vi "Sequence.Test.NextStep.vi"(8 "error in":errorcluster, 11 "Data in":T7={"BeginTS"=timestamp(0 s since 1904-01-01), "EndTS"=timestamp(0 s since 1904-01-01), "State"=enum."Init", "Status.Work"=enum."-", "Status.Process"=enum."-", "Status.Home"=enum."-", "Status.Wabco"=enum."-", "Status.Client"=enum."-", "BreakReason"=enum."-", "BreakSource"=enum."-", "DoorLock"=FALSE, "Status.Prod"=[], "UserAction"={"Stop"=FALSE, "Pause"=FALSE, "Next"=FALSE}, "UserData"={"GuiMode"=enum."Process", "Test"={"IgnoreResults"=FALSE, "IgnoreImages"=FALSE, "ServiceMode"=FALSE}, "ContinueOrder"=FALSE}, "Error"={"status"=FALSE, "code"=0, "source"=""}, "Code"={"Ready"=FALSE, "DoubleOrder"=FALSE, "OrderDone"=FALSE, "AllowSingleSlot"=FALSE, "CheckDM"=FALSE, "ThresholdA"=0, "ThresholdB"=0, "Plate"=enum."Wabco", "ImgPath"=path "", "Variant"={"State"=enum."Init", "ImgPath"=path "", "WabcoPlate"="", "WabcoProduct"="", "ClientProduct"="", "ClientPlate"="", "TotalQuantity"=0, "OrderQuantity"=0, "Serial"=0, "Wabco"={"LaserJob"="", "AdditionalTxt"="037", "FactoryCode"="", "RevID"=0, "ForkID"=0, "FailuresLimit"=0, "GlobalCnt"=0, "ScannerProgram"=0, "SerialFormat"=enum."6 dig", "CoordA"={"X"=0.0, "Y"=0.0, "Angle"=0.0}, "CoordB"={"X"=0.0, "Y"=0.0, "Angle"=0.0}, "DMCconfig"=0}, "Client"={"LaserJob"="", "AdditionalTxt"="", "FactoryCode"="037", "RevID"=0, "ForkID"=0, "FailuresLimit"=0, "GlobalCnt"=0, "ScannerProgram"=0, "SerialFormat"=enum."6 dig", "CoordA"={"X"=0.0, "Y"=0.0, "Angle"=0.0}, "CoordB"={"X"=0.0, "Y"=0.0, "Angle"=0.0}, "DMCconfig"=0}}}, "Rotations"=0, "ProdIdx"=0, "ProdDone"=[], "PrintedSerials-Wabco"=[], "PrintedSerials-Client"=[], "Counters-Wabco"={"Expected"=0, "Done"=0, "OK"=0, "NOK"=0, "NOKlimit"=0, "Part"=0, "PartOK"=0}, "Counters-Client"={"Expected"=0, "Done"=0, "OK"=0, "NOK"=0, "NOKlimit"=0, "Part"=0, "PartOK"=0}}) -> (0 "error out":errorcluster, 2 "Final Status":T5, 3 "Data out":T7={"BeginTS"=timestamp(0 s since 1904-01-01), "EndTS"=timestamp(0 s since 1904-01-01), "State"=enum."Init", "Status.Work"=enum."-", "Status.Process"=enum."-", "Status.Home"=enum."-", "Status.Wabco"=enum."-", "Status.Client"=enum."-", "BreakReason"=enum."-", "BreakSource"=enum."-", "DoorLock"=FALSE, "Status.Prod"=[], "UserAction"={"Stop"=FALSE, "Pause"=FALSE, "Next"=FALSE}, "UserData"={"GuiMode"=enum."Process", "Test"={"IgnoreResults"=FALSE, "IgnoreImages"=FALSE, "ServiceMode"=FALSE}, "ContinueOrder"=FALSE}, "Error"={"status"=FALSE, "code"=0, "source"=""}, "Code"={"Ready"=FALSE, "DoubleOrder"=FALSE, "OrderDone"=FALSE, "AllowSingleSlot"=FALSE, "CheckDM"=FALSE, "ThresholdA"=0, "ThresholdB"=0, "Plate"=enum."Wabco", "ImgPath"=path "", "Variant"={"State"=enum."Init", "ImgPath"=path "", "WabcoPlate"="", "WabcoProduct"="", "ClientProduct"="", "ClientPlate"="", "TotalQuantity"=0, "OrderQuantity"=0, "Serial"=0, "Wabco"={"LaserJob"="", "AdditionalTxt"="037", "FactoryCode"="", "RevID"=0, "ForkID"=0, "FailuresLimit"=0, "GlobalCnt"=0, "ScannerProgram"=0, "SerialFormat"=enum."6 dig", "CoordA"={"X"=0.0, "Y"=0.0, "Angle"=0.0}, "CoordB"={"X"=0.0, "Y"=0.0, "Angle"=0.0}, "DMCconfig"=0}, "Client"={"LaserJob"="", "AdditionalTxt"="", "FactoryCode"="037", "RevID"=0, "ForkID"=0, "FailuresLimit"=0, "GlobalCnt"=0, "ScannerProgram"=0, "SerialFormat"=enum."6 dig", "CoordA"={"X"=0.0, "Y"=0.0, "Angle"=0.0}, "CoordB"={"X"=0.0, "Y"=0.0, "Angle"=0.0}, "DMCconfig"=0}}}, "Rotations"=0, "ProdIdx"=0, "ProdDone"=[], "PrintedSerials-Wabco"=[], "PrintedSerials-Client"=[], "Counters-Wabco"={"Expected"=0, "Done"=0, "OK"=0, "NOK"=0, "NOKlimit"=0, "Part"=0, "PartOK"=0}, "Counters-Client"={"Expected"=0, "Done"=0, "OK"=0, "NOK"=0, "NOKlimit"=0, "Part"=0, "PartOK"=0}})   [LabVIEW 2016]
uses:
  Sequence.Data.ctl
  Sequence.State.ctl
  Sequence.Step.Status.ctl
  Sequence.Test.BreakReason.ctl
  Sequence.Test.BreakSource.ctl
  Sequence.Test.Status.ctl
  Sequence.Slot.StatusData.ctl
  Sequence.Test.Unload.Status.ctl
  Sequence.Prod.StatusData.ctl
  Sequence.UserActions.ctl
  Sequence.UserData.ctl
  Sequence.MainMode.ctl
  Gui/MainGui.TestOptions.ctl
  Sequence.Code.Sets.ctl
  Sequence.PlateType.ctl
  Logger/Logger.Variant.Sets.ctl
  Station/Station.Changeover.State.vi
  Station/Station.Plate.Properties.ctl
  Sequence.Code.SerialFormat.ctl
  Drivers/V7310/LowLevel/V7310.Job.Sets.ctl
  Sequence.Counters.ctl
  Drivers/FestoCPX/Station/FestoCPX.Station.ProdArmPosition.ctl
panel:
  out "element":T1
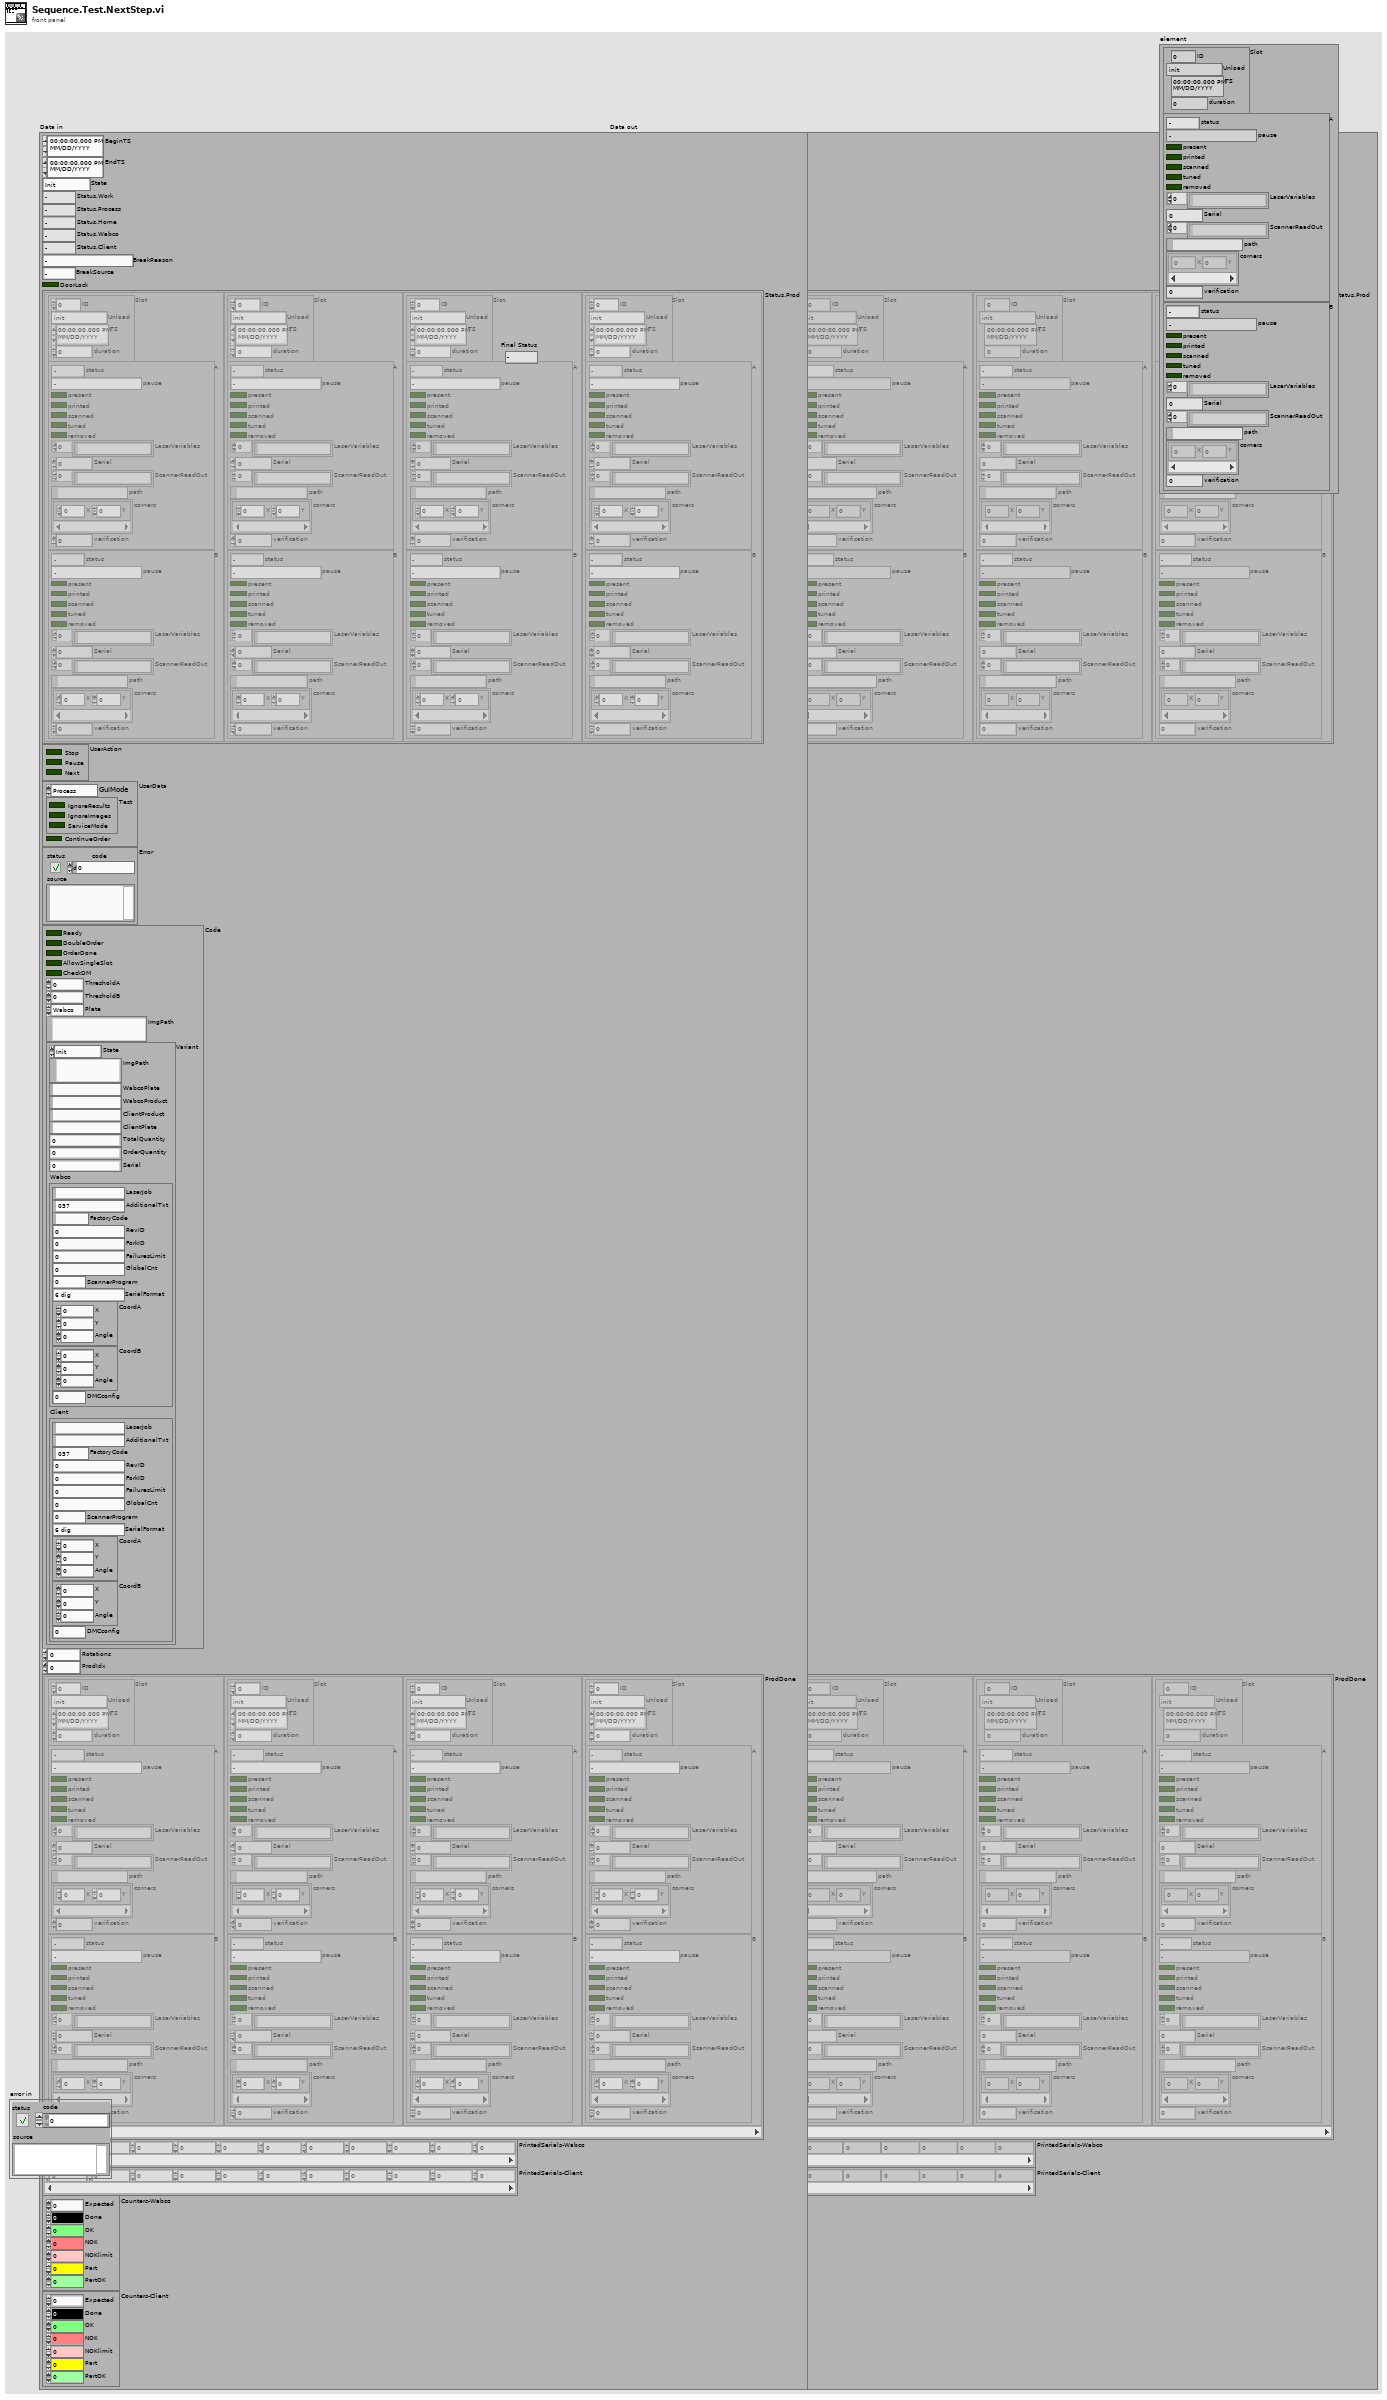
[diagram p1: front panel]
types:
  T1 = typedef "Sequence.Test.Status.ctl" = cluster{"Slot":T2, "A":T4, "B":T4}
  T2 = typedef "Sequence.Slot.StatusData.ctl" = cluster{"ID":i32, "Unload":T3, "TS":timestamp, "duration":u32}
  T3 = typedef "Sequence.Test.Unload.Status.ctl" = enum16{"init", "check NOK", "check OK", "wait on NOK", "wait on OK", "wait on Unload", "done"}
  T4 = typedef "Sequence.Prod.StatusData.ctl" = cluster{"status":T5, "pause":T6, "present":bool, "printed":bool, "scanned":bool, "tuned":bool, "removed":bool, "LaserVariables":string[], "Serial":i32, "ScannerReadOut":string[], "path":path, "corners":cluster{"X":i32, "Y":i32}[], "verification":u8}
  T5 = typedef "Sequence.Step.Status.ctl" = enum16{"-", "Pending", "Running", "Skipped", "Passed", "Failed", "Done", "Error", "Aborted", "Stopped"}
  T6 = typedef "Sequence.Test.BreakReason.ctl" = enum16{"-", "NOK container", "OK container", "Rev empty", "Rev missing", "Rev wrong", "Fork missing", "Fork wrong", "NOK limit", "Unload failure", "Single slot", "Part done", "Err: Prod move work", "Err: Prod move home", "Err: Prod lift work", "Err: Prod lift home", "Err: Prod Arm Work", "Err: Prod Arm NOK", "Err: Prod Arm OK", "Err: Prod NOK suck", "Err: Prod NOK drop", "Err: Prod OK missing", "Err: Prod OK suck", "Err: Prod OK drop"}
  T7 = typedef "Sequence.Data.ctl" = cluster{"BeginTS":timestamp, "EndTS":timestamp, "State":T8, "Status.Work":T5, "Status.Process":T5, "Status.Home":T5, "Status.Wabco":T5, "Status.Client":T5, "BreakReason":T6, "BreakSource":T9, "DoorLock":bool, "Status.Prod":T1[], "UserAction":T10, "UserData":T11, "Error":errorcluster, "Code":T14, "Rotations":i32, "ProdIdx":i32, "ProdDone":T1[], "PrintedSerials-Wabco":i32[], "PrintedSerials-Client":i32[], "Counters-Wabco":T21, "Counters-Client":T21}
  T8 = typedef "Sequence.State.ctl" = enum16{"Init", "Idle", "Home", "Work", "Run", "Pause"}
  T9 = typedef "Sequence.Test.BreakSource.ctl" = enum16{"-", "A", "B", "A/B"}
  T10 = typedef "Sequence.UserActions.ctl" = cluster{"Stop":bool, "Pause":bool, "Next":bool}
  T11 = typedef "Sequence.UserData.ctl" = cluster{"GuiMode":T12, "Test":T13, "ContinueOrder":bool}
  T12 = typedef "Sequence.MainMode.ctl" = enum16{"Process", "Base", "Order", "Manual", "Logs", "Results", "Stats", "DMC Config"}
  T13 = typedef "MainGui.TestOptions.ctl" = cluster{"IgnoreResults":bool, "IgnoreImages":bool, "ServiceMode":bool}
  T14 = typedef "Sequence.Code.Sets.ctl" = cluster{"Ready":bool, "DoubleOrder":bool, "OrderDone":bool, "AllowSingleSlot":bool, "CheckDM":bool, "ThresholdA":u8, "ThresholdB":u8, "Plate":T15, "ImgPath":path, "Variant":T16}
  T15 = typedef "Sequence.PlateType.ctl" = enum16{"Wabco", "Client"}
  T16 = typedef "Logger.Variant.Sets.ctl" = cluster{"State":T17, "ImgPath":path, "WabcoPlate":string, "WabcoProduct":string, "ClientProduct":string, "ClientPlate":string, "TotalQuantity":u16, "OrderQuantity":u16, "Serial":i32, "Wabco":T18, "Client":T18}
  T17 = typedef "Station.Changeover.State.vi" = enum16{"Init", "Scaning", "NOK", "Wait for ack", "Ready"}
  T18 = typedef "Station.Plate.Properties.ctl" = cluster{"LaserJob":string, "AdditionalTxt":string, "FactoryCode":string, "RevID":u8, "ForkID":u8, "FailuresLimit":u16, "GlobalCnt":i32, "ScannerProgram":u8, "SerialFormat":T19, "CoordA":T20, "CoordB":T20, "DMCconfig":i32}
  T19 = typedef "Sequence.Code.SerialFormat.ctl" = enum8{"", "6 dig", "7 dig"}
  T20 = typedef "V7310.Job.Sets.ctl" = cluster{"X":dbl, "Y":dbl, "Angle":dbl}
  T21 = typedef "Sequence.Counters.ctl" = cluster{"Expected":u16, "Done":u16, "OK":u16, "NOK":u16, "NOKlimit":u16, "Part":u16, "PartOK":u16}
  T22 = typedef "Sequence.SerialsFglb.StatusFlags.ctl" = cluster{"Global":bool, "NokLimit":bool, "PartDone":bool, "Completed":bool}
  T23 = typedef "FestoCPX.Station.ProdArmPosition.ctl" = enum16{"Work", "OK", "NOK"}
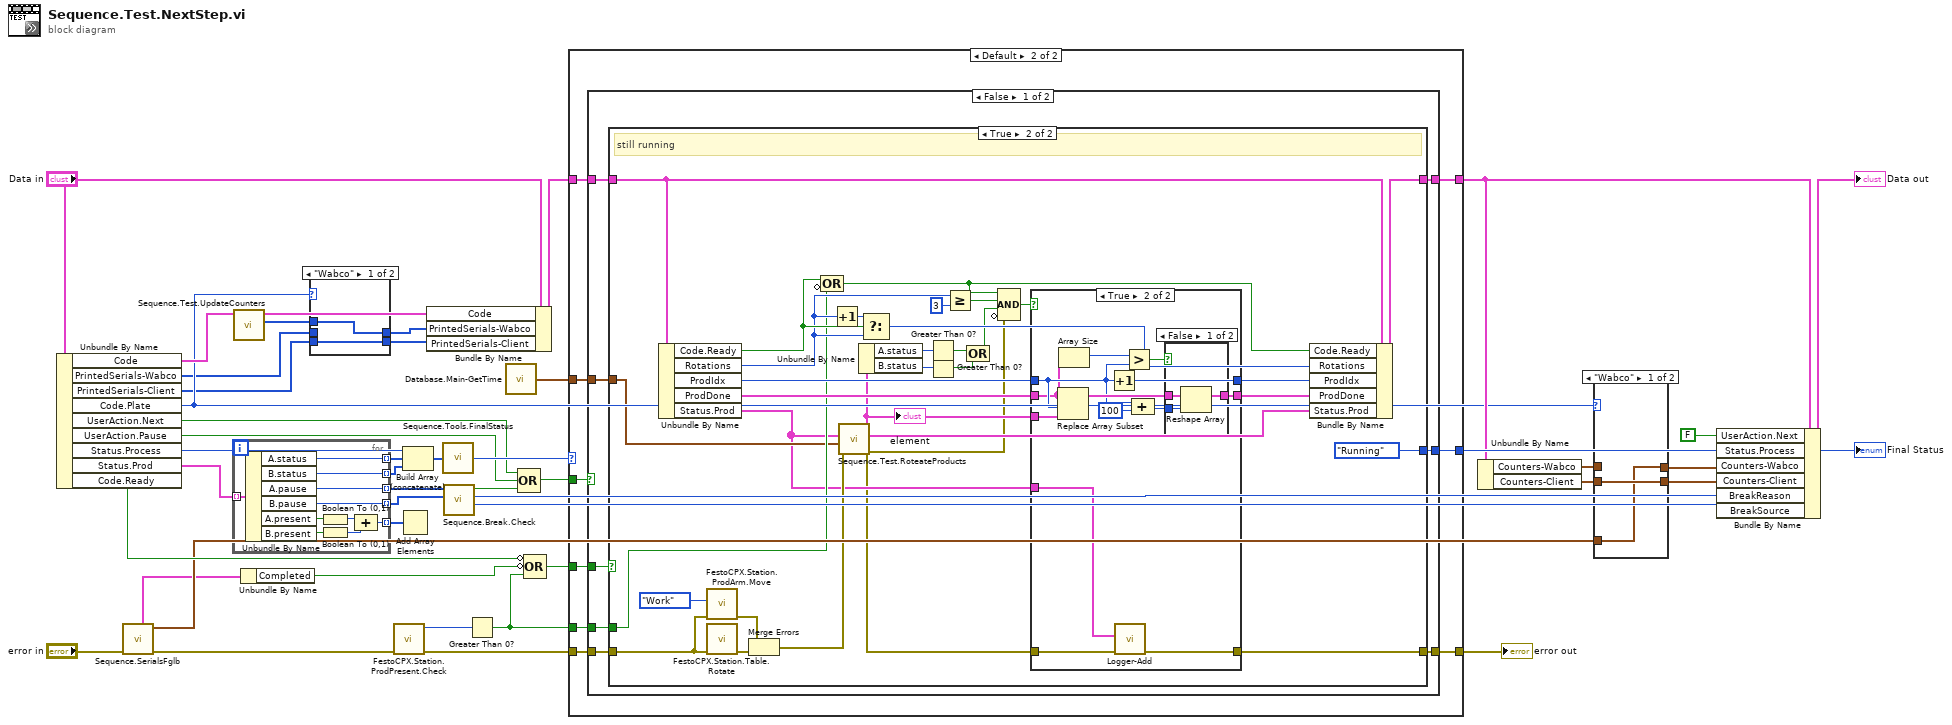
[diagram p0: block diagram]
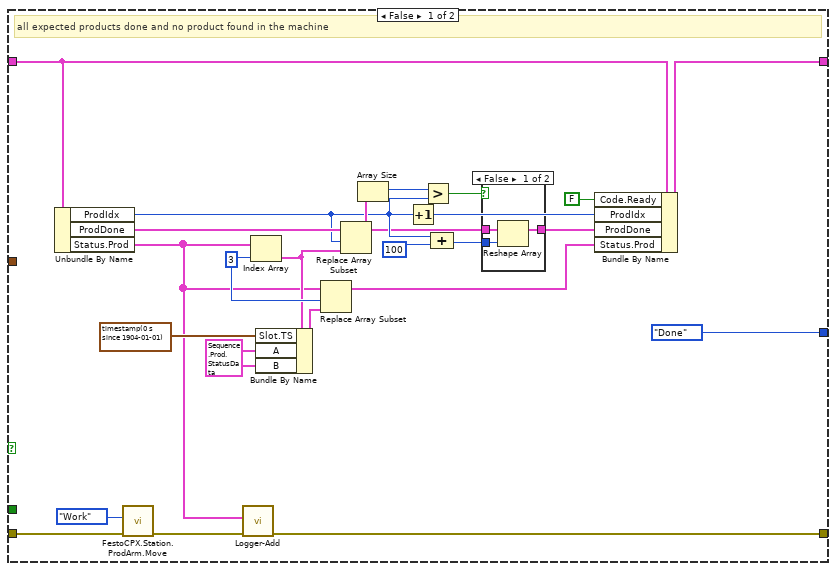
[diagram p5: hidden frame]
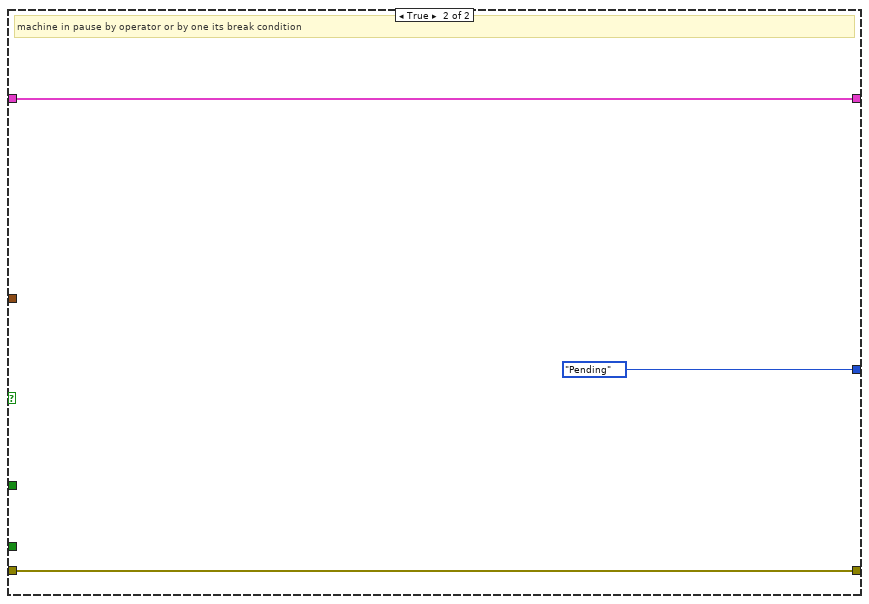
[diagram p9: hidden frame]
diagram:
  n1 = Unbundle By Name("Data in") -> ("Code"=w11:T14, "PrintedSerials-Wabco"=w9:i32[], "PrintedSerials-Client"=w8:i32[], "Code.Plate"=w10:T15, "UserAction.Next"=w28:bool, "UserAction.Pause"=w35:bool, "Status.Process"=w33:T5, "Status.Prod"=w6:T1[], "Code.Ready"=w29:bool)
  n2 = call "Sequence.SerialsFglb.vi"("error in"="error in") -> ("error out"=w17:errorcluster, "Counters out"=w22:T21, "StatusFlags"=w20:T22)  [unwired: 6 in, 2 out]
  n3 = for {
    tunnel: w6 -> [w53] mode=indexing
    tunnel: [w55] -> w45 mode=indexing
    tunnel: [w54] -> w31 mode=indexing
    tunnel: [w52] -> w41 mode=indexing
    tunnel: [w51] -> w40 mode=indexing
    tunnel: [w46] -> w18 mode=indexing
    n4 = Unbundle By Name(w53) -> ("A.status"=w55:T5, "B.status"=w54:T5, "A.pause"=w52:T6, "B.pause"=w51:T6, "A.present"=w49:bool, "B.present"=w50:bool)
    n5 = Boolean To (0,1)(Boolean=w49) -> (0, 1=w48:i16)
    n6 = Boolean To (0,1)(Boolean=w50) -> (0, 1=w47:i16)
    n7 = Compound Arithmetic op=ADD(w48, w47) -> (w46:i16)
  }
  n8 = call "Sequence.Test.UpdateCounters.vi"("Code in"=w11) -> ("Printed serials out"=w7:i32[], "Code out"=w5:T14)  [unwired: 8 in, 1 out]
  n9 = Unbundle By Name(w20) -> ("Completed"=w19:bool)
  n10 = case shown="\"Wabco\"" w10 {
    tunnel: w7 -> [w56 w59]
    tunnel: w8 -> [w57 _]
    tunnel: [w57 w59] -> w3
    tunnel: [w56 w58] -> w4
    tunnel: w9 -> [_ w58]
    frame "Wabco" {
    }
    frame "Client" {
    }
  }
  n11 = call "FestoCPX.Station.ProdPresent.Check.vi"("error in"=w17) -> ("error out"=w16:errorcluster, "#products in the machine"=w15:i32)  [unwired: 5 in, 4 out]
  n12 = Add Array Elements(numeric array=w18) -> ()  [unwired: 1 out]
  n13 = Build Array (concatenate)(w33, w45, w31) -> (w44:T5[])
  n14 = Bundle By Name(cluster="Data in", "Code"=w5, "PrintedSerials-Wabco"=w4, "PrintedSerials-Client"=w3) -> (w1:T7)
  n15 = call "Sequence.Tools.FinalStatus.vi"("Status array"=w44) -> ("Final Status"=w43:T5)
  n16 = call "Sequence.Break.Check.vi"("Pauses B"=w40, "Pauses A"=w41) -> ("break source"=w13:T9, "break reason"=w12:T6, "break found"=w36:bool)  [unwired: 7 in]
  n17 = Greater Than 0?(x=w15) -> (x > 0?=w30:bool)
  n18 = call "Database.Main-GetTime.vi"() -> ("TS"=w14:timestamp)  [unwired: 1 in]
  n19 = Compound Arithmetic op=OR(w28, w35, w36) -> (w34:bool)
  n20 = Compound Arithmetic op=OR(invert w29, invert w19, w30) -> (w39:bool)
  n21 = case shown="Default" w43 {
    selector: w43 -> [w60 _]
    tunnel: w1 -> [w62 w71]
    tunnel: [w62 w70] -> w27
    tunnel: w16 -> [w61 w69]
    tunnel: [w61 w68] -> w42
    tunnel: [w60 w67] -> w32
    tunnel: w39 -> [_ w66]
    tunnel: w34 -> [_ w65]
    tunnel: w30 -> [_ w64]
    tunnel: w14 -> [_ w63]
    frame "Error".."Stopped" {
      # "machine stopped, error or aborted"
    }
    frame Default {
      n22 = case shown="False" w65 {
        tunnel: w71 -> [w79 w161]
        tunnel: [w74 w161] -> w70
        tunnel: w69 -> [w78 w160]
        tunnel: [w73 w160] -> w68
        tunnel: [w76 Sequence.Step.Status."Pending" ("Final Status")] -> w67
        tunnel: w66 -> [w77 _]
        tunnel: w64 -> [w75 _]
        tunnel: w63 -> [w72 _]
        frame False {
          n23 = case shown="True" w77 {
            tunnel: w79 -> [w102 w138]
            tunnel: [w101 w137] -> w74
            tunnel: w78 -> [w93 w126]
            tunnel: [w100 w131] -> w73
            tunnel: [Sequence.Step.Status."Done" ("Final Status") Sequence.Step.Status."Running" ("Final Status")] -> w76
            tunnel: w75 -> [_ w112]
            tunnel: w72 -> [_ w110]
            frame False {
              w88 = T4 {"status"=enum."-", "pause"=enum."-", "present"=FALSE, "printed"=FALSE, "scanned"=FALSE, "tuned"=FALSE, "removed"=FALSE, "LaserVariables"=[], "Serial"=0, "ScannerReadOut"=[], "path"=path "", "corners"=[], "verification"=0} ("A")
              w91 = 3 ("index")
              # "all expected products done and no product found in the machine"
              n24 = Unbundle By Name(w102) -> ("ProdIdx"=w96:i32, "ProdDone"=w99:T1[], "Status.Prod"=w80:T1[])
              n25 = call "FestoCPX.Station.ProdArm.Move.vi"("error in"=w93, "Product Status"=FestoCPX.Station.ProdArmPosition."Work") -> ("error out"=w92:errorcluster)  [unwired: 9 in]
              n26 = call "Logger-Add.vi"("error in"=w92, "All Slots"=w80) -> ("error out"=w100:errorcluster)  [unwired: 9 in]
              n27 = Index Array(array=w80, index=w91) -> (element=w82:T1)
              n28 = Bundle By Name(cluster=w82, "Slot.TS"=timestamp(0 s since 1904-01-01) ("Slot.TSto"), "A"=w88, "B"=w88) -> (w90:T1)
              n29 = Replace Array Subset(array=w80, new element=w90, index=w91) -> (w89:T1[])
              n30 = Replace Array Subset(array=w99, new element=w82, index=w96) -> (w84:T1[])
              n31 = Array Size(array=w99) -> (size(s)=w83:i32)
              n32 = Increment(x=w96) -> (x+1=w97:i32)
              n33 = Greater?(x=w83, y=w97) -> (0:w85:bool)
              n34 = Compound Arithmetic op=ADD(w97, 100 ("value")) -> (w87:i32)
              n35 = case shown="False" w85 {
                tunnel: w84 -> [w106 w107]
                tunnel: w87 -> [w105 _]
                tunnel: [w104 w107] -> w98
                frame False {
                  n36 = Reshape Array(w106, w105) -> (w104:T1[])
                }
                frame True {
                }
              }
              n37 = Bundle By Name(cluster=w102, "Code.Ready"=FALSE, "ProdIdx"=w97, "ProdDone"=w98, "Status.Prod"=w89) -> (w101:T7)
            }
            frame True {
              # "still running"
              n38 = Unbundle By Name(w138) -> ("Code.Ready"=w124:bool, "Rotations"=w123:i32, "ProdIdx"=w117:i32, "ProdDone"=w118:T1[], "Status.Prod"=w109:T1[])
              n39 = call "FestoCPX.Station.ProdArm.Move.vi"("error in"=w126, "Product Status"=FestoCPX.Station.ProdArmPosition."Work") -> ("error out"=w125:errorcluster)  [unwired: 9 in]
              n40 = call "FestoCPX.Station.Table.Rotate.vi"("error in"=w126) -> ("error out"=w132:errorcluster)  [unwired: 10 in]
              n41 = Merge Errors(w125, w132) -> (w111:errorcluster)
              n42 = Compound Arithmetic op=OR(w124, invert w112) -> (w115:bool)
              n43 = Increment(x=w123) -> (x+1=w128:i32)
              n44 = call "Sequence.Test.RoteateProducts.vi"("error in (no error)"=w111, "TS"=w110, "Status.Prod in"=w109) -> ("error out"=w108:errorcluster, "Status.Prod out"=w114:T1[], "Status Prev"=w116:T1)  [unwired: 6 in]
              "element" <- w116
              n45 = Unbundle By Name(w116) -> ("A.status"=w122:T5)  [unwired: 1 out]
              n46 = Select(t=w128, s=w124, f=w123) -> (s? t:f=w127:i32)
              n47 = Greater Than 0?(x=w122) -> (x > 0?=w121:bool)
              n48 = Greater Than 0?(x=w122) -> (x > 0?=w120:bool)
              n49 = Greater Or Equal?(x=w123, y=3) -> (x >= y?=w133:bool)
              n50 = Compound Arithmetic op=OR(w121, w120) -> (w119:bool)
              n51 = Compound Arithmetic op=AND(w115, w133, w119, invert w108) -> (w130:bool)
              n52 = case shown="True" w130 {
                tunnel: w118 -> [w140 w147]
                tunnel: [w140 w150] -> w113
                tunnel: w116 -> [_ w143]
                tunnel: w117 -> [w141 w149]
                tunnel: [w141 w148] -> w135
                tunnel: w108 -> [w139 w145]
                tunnel: [w139 w144] -> w131
                tunnel: w109 -> [_ w142]
                frame False {
                }
                frame True {
                  n53 = Replace Array Subset(array=w147, new element=w143, index=w149) -> (w151:T1[])
                  n54 = Array Size(array=w147) -> (size(s)=w146:i32)
                  n55 = Increment(x=w149) -> (x+1=w148:i32)
                  n56 = call "Logger-Add.vi"("error in"=w145, "All Slots"=w142) -> ("error out"=w144:errorcluster)  [unwired: 9 in]
                  n57 = Greater?(x=w146, y=w148) -> (0:w152:bool)
                  n58 = Compound Arithmetic op=ADD(w148, 100 ("value")) -> (w154:i32)
                  n59 = case shown="False" w152 {
                    tunnel: w151 -> [w157 w158]
                    tunnel: w154 -> [w156 _]
                    tunnel: [w155 w158] -> w150
                    frame False {
                      n60 = Reshape Array(w157, w156) -> (w155:T1[])
                    }
                    frame True {
                    }
                  }
                }
              }
              n61 = Bundle By Name(cluster=w138, "Code.Ready"=w115, "Rotations"=w127, "ProdIdx"=w135, "ProdDone"=w113, "Status.Prod"=w114) -> (w137:T7)
            }
          }
        }
        frame True {
          # "machine in pause by operator or by one its break condition"
        }
      }
    }
  }
  "error out" <- w42
  "Final Status" <- w32
  n62 = Unbundle By Name(w27) -> ("Counters-Wabco"=w26:T21, "Counters-Client"=w24:T21)
  n63 = case shown="\"Wabco\"" w10 {
    tunnel: w26 -> [_ w165]
    tunnel: [w162 w165] -> w25
    tunnel: [w163 w164] -> w23
    tunnel: w24 -> [w163 _]
    tunnel: w22 -> [w162 w164]
    frame "Wabco" {
    }
    frame "Client" {
    }
  }
  n64 = Bundle By Name(cluster=w27, "UserAction.Next"=FALSE, "Status.Process"=w32, "Counters-Wabco"=w25, "Counters-Client"=w23, "BreakReason"=w12, "BreakSource"=w13) -> (→"Data out":T7)
